vi "TEST_Menu.vi"() -> ()   [LabVIEW 2021]
uses:
  <vilib>/Utility/miscctls.llb/LVMenuShortCut.ctl
  Menu.lvclass
  MenuSelection.ctl
  Picture2D/src/Color/Color.lvclass
  Picture2D/src/2DPictureControl/2DPictureControl.lvclass
  <vilib>/Utility/miscctls.llb/LVPointTypeDef.ctl
  91be992c-c2ba-4221-a176-dbd6ab68e1f9.vi
  Picture2D/src/Picture/Image.lvclass
  C:/GitHub/Picture2D/src/IDrawable/IDrawable.lvclass
  SetBackgroundColor.vi
  SetBorderColor.vi
  SetHiliteColor.vi
  SetHiliteTextColor.vi
  SetTextColor.vi
  <vilib>/ErrorRing/Error Ring.xnode
panel:
  out "enabled":bool
  out "2D Picture out":picture
  in  "Color Theme":enum16{"LabVIEW", "Dark"}(ring)
  out "item name":string
  out "submenu tags":string[](array[string])
  out "checked":bool
  out "short cut":T1
  out "2D Picture":picture
  out "ItemPath":string
  out "ItemTag":string
  out "error out":errorcluster
  out "item tags out":string[](array[string])
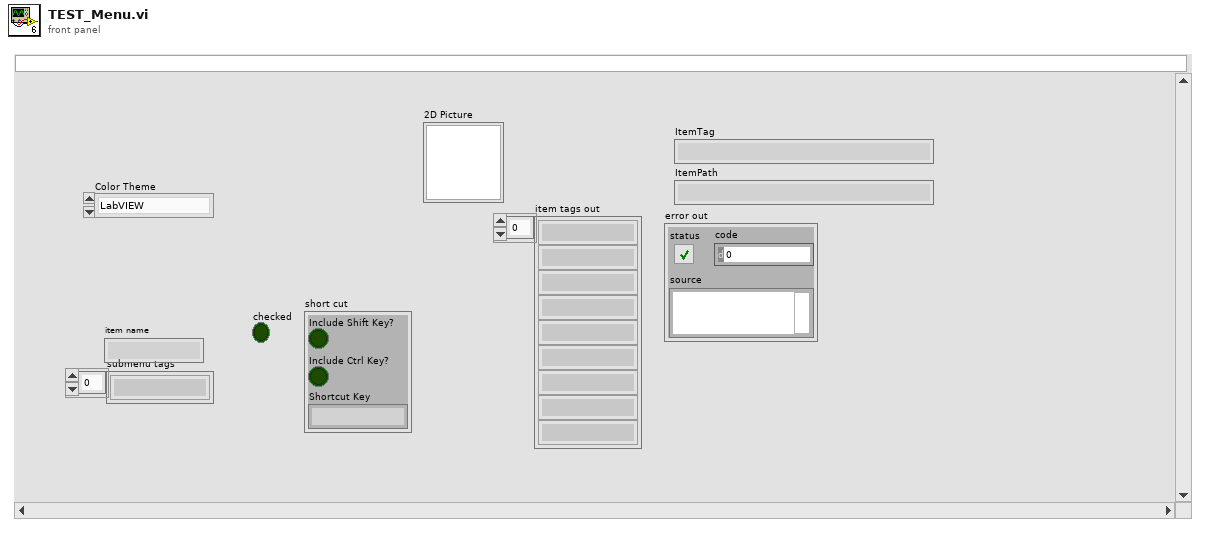
[diagram p1: front panel]
types:
  T1 = typedef "LVMenuShortCut.ctl" = cluster{"Include Shift Key?":bool, "Include Ctrl Key?":bool, "Shortcut Key":string}
  T2 = enum16{"Init Menu", "Init Menu Icon", "Execute", "Close"}
  T3 = enum16{"Init Menu", "Init Menu Icon", "Execute", "Close"}[]
  T4 = typedef "LVPointTypeDef.ctl" = cluster{"Horizontal":i16, "Vertical":i16}
  T5 = typedef "LVBoundsTypeDef.ctl" = cluster{"Width":u32, "Height":u32}
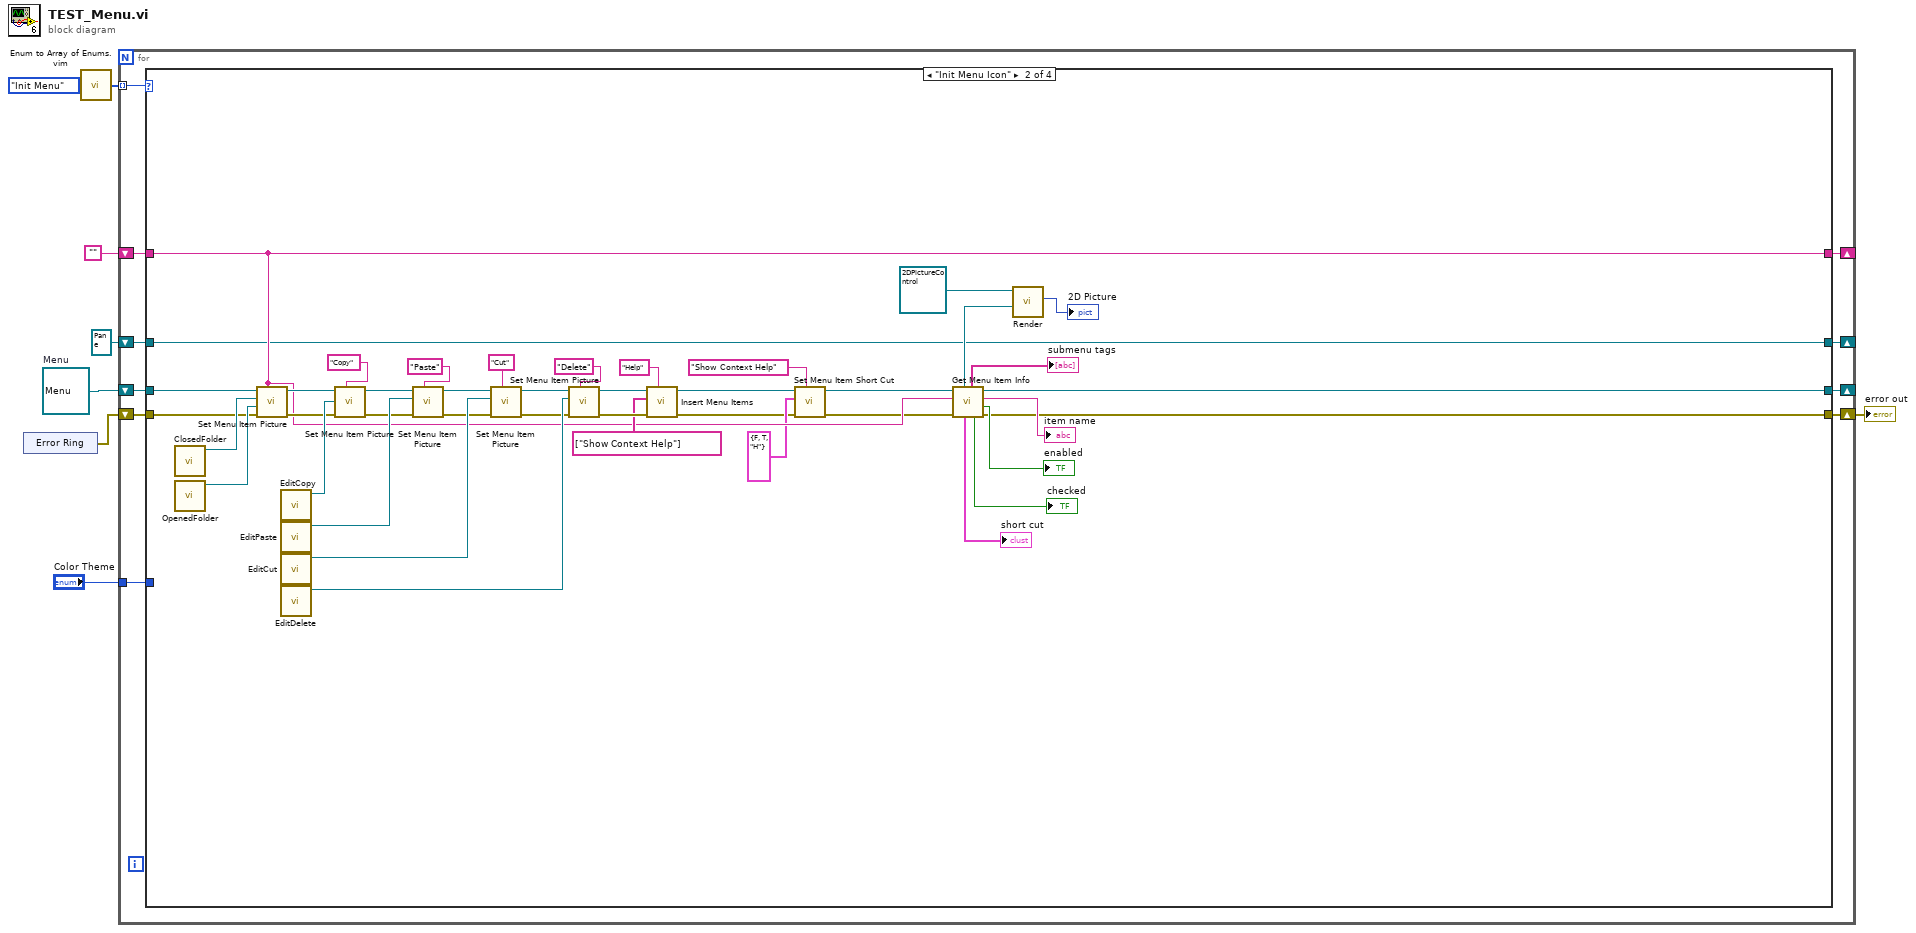
[diagram p0: block diagram]
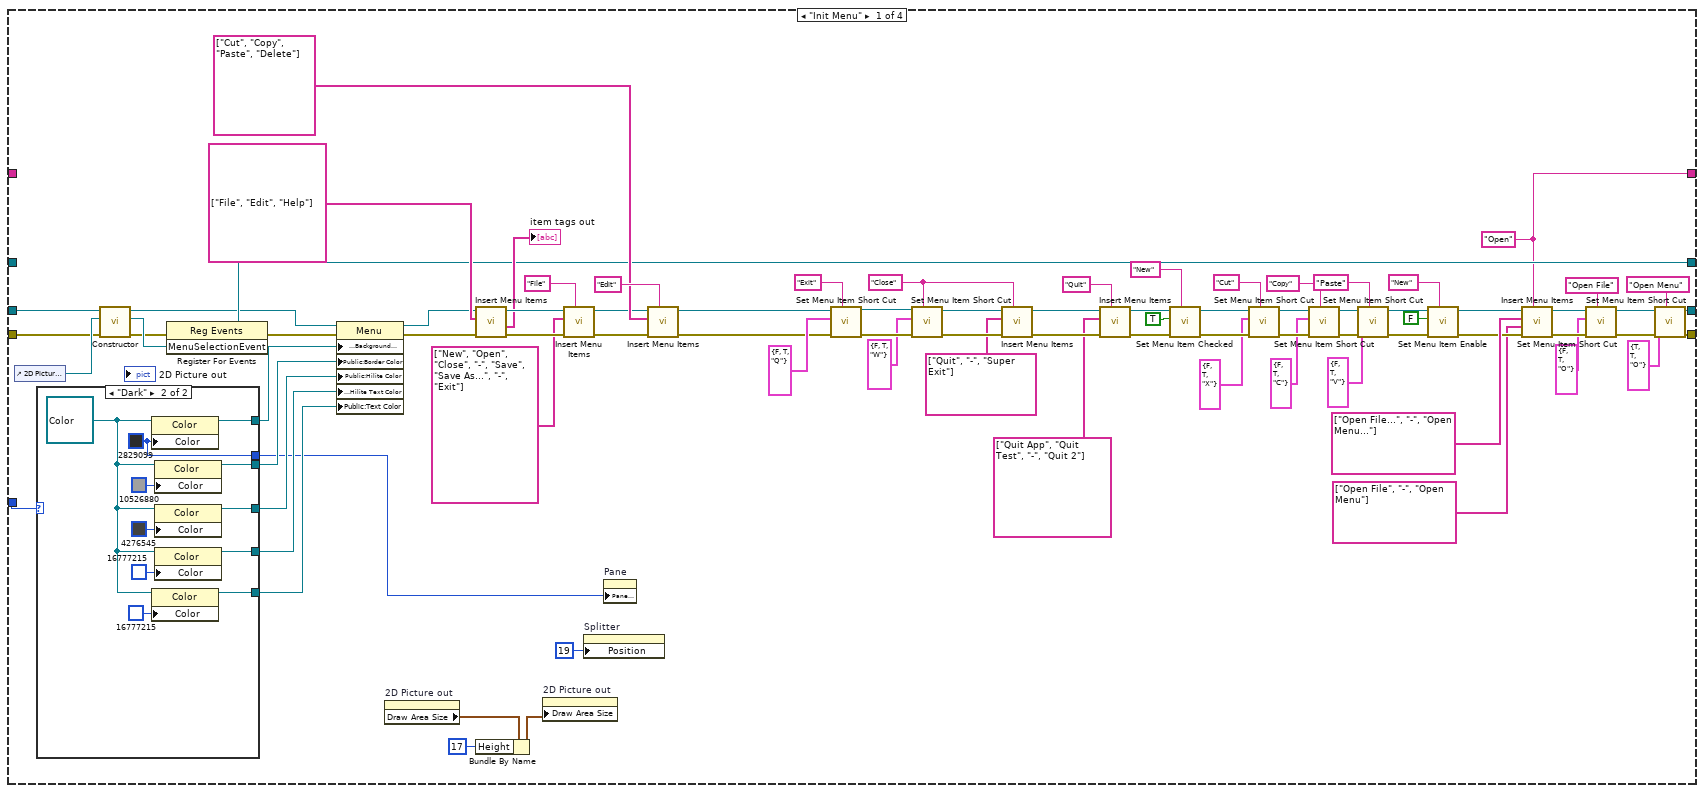
[diagram p2: hidden frame]
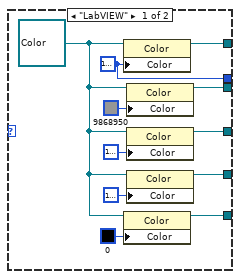
[diagram p3: hidden frame]
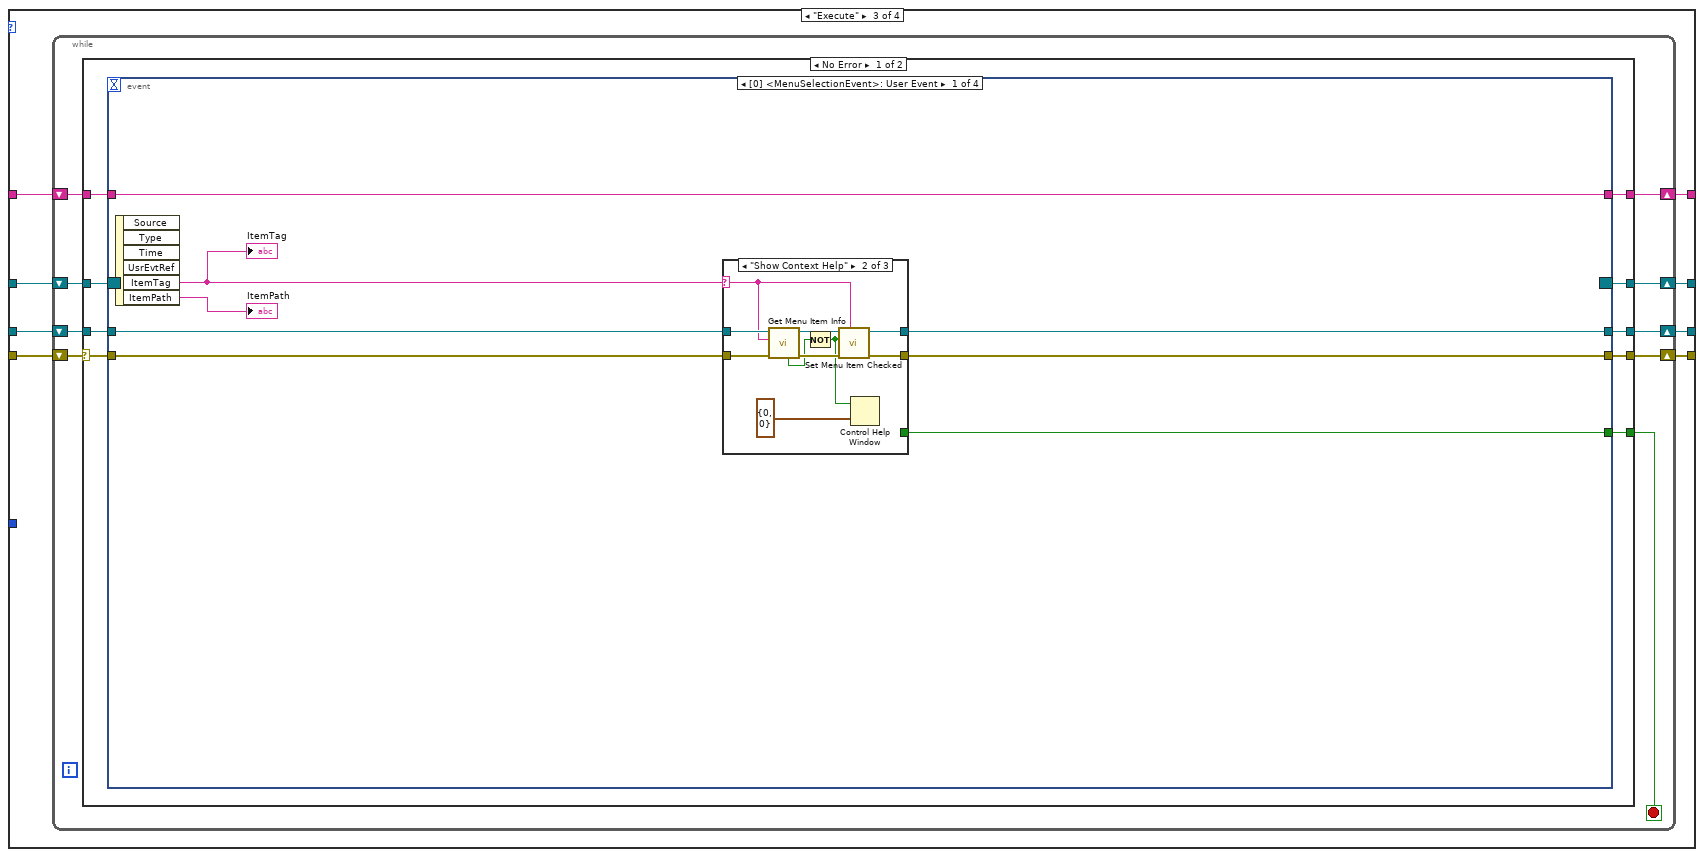
[diagram p4: hidden frame]
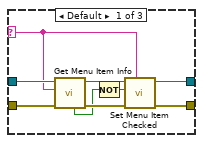
[diagram p5: hidden frame]
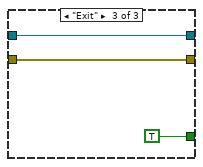
[diagram p6: hidden frame]
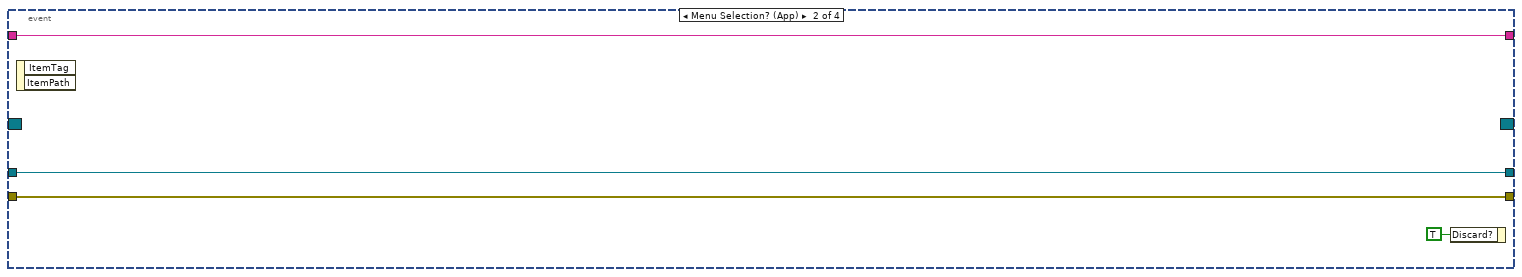
[diagram p7: hidden frame]
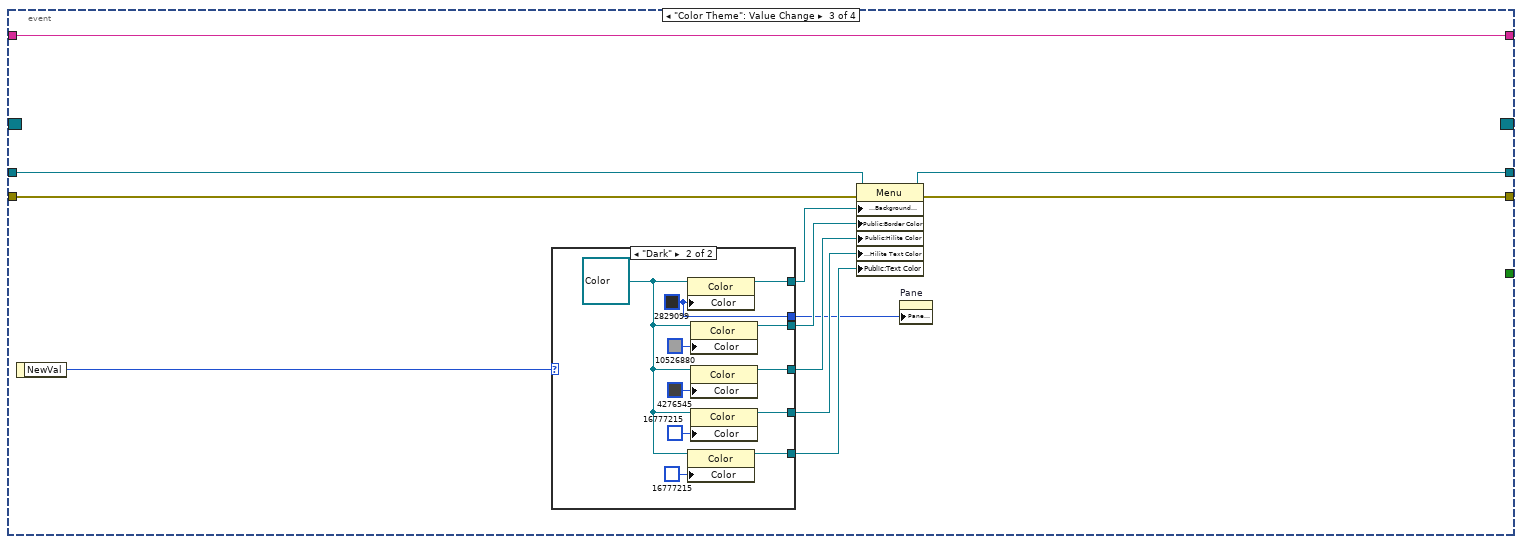
[diagram p8: hidden frame]
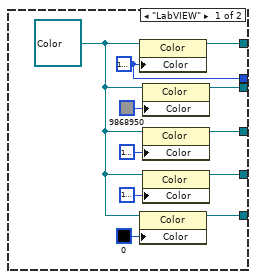
[diagram p9: hidden frame]
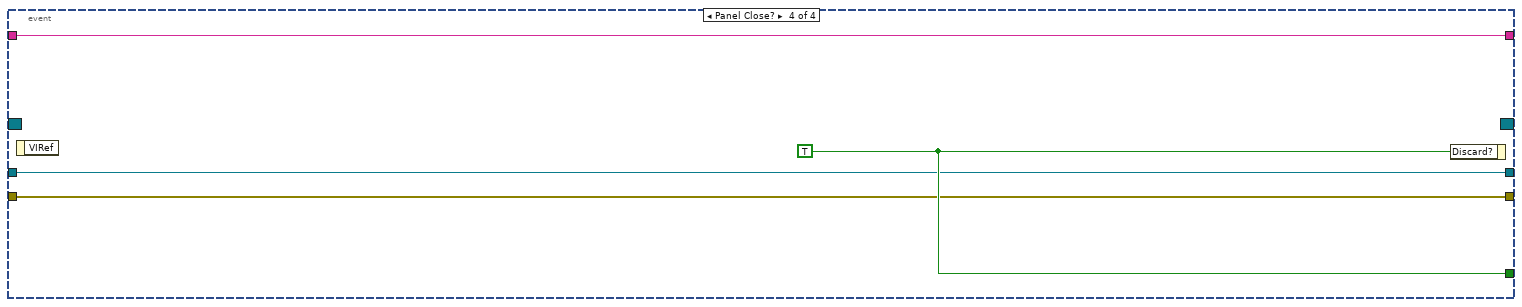
[diagram p10: hidden frame]
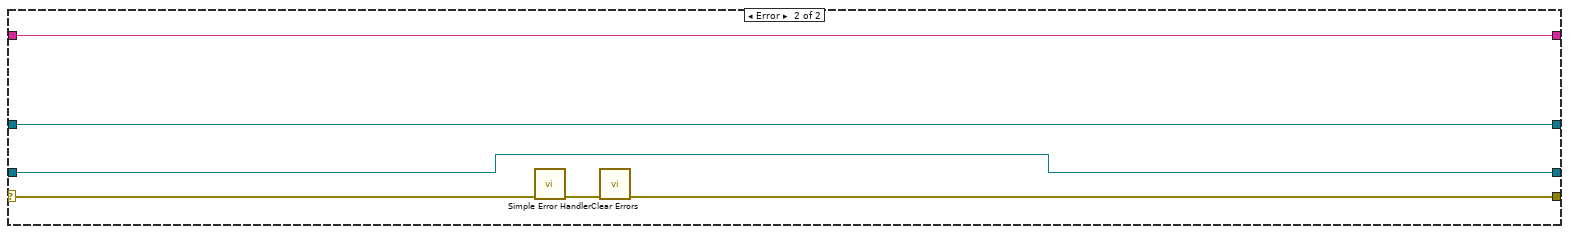
[diagram p11: hidden frame]
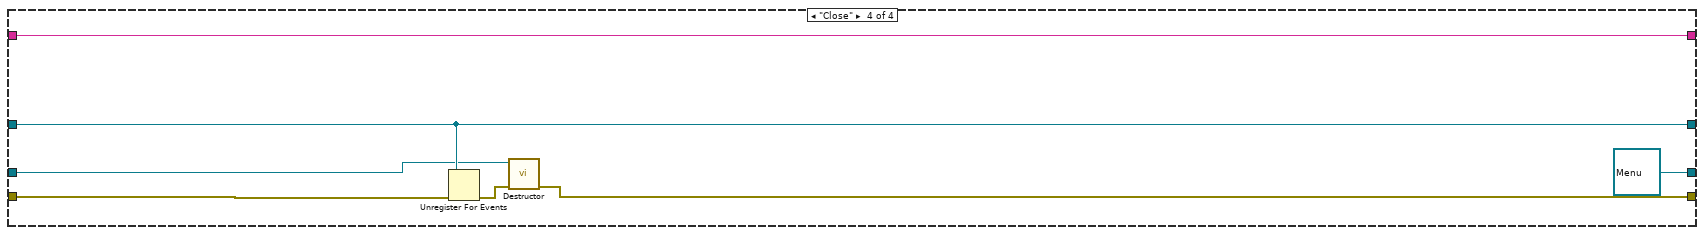
[diagram p12: hidden frame]
diagram:
  w8 = refnum<class "Menu.lvclass"> refnum  # Menu
  n1 = xnode "Error Ring"() -> ("error out"=w4:errorcluster)
  n2 = call "Enum to Array of Enums.vim"("enum"=T2."Init Menu") -> ("array of enums"=w5:T3)
  n3 = for {
    tunnel: "Color Theme" -> [w16]
    shift-right: [w15] -> _
    shift-left: w8 -> [w18]
    tunnel: w5 -> [w12] mode=indexing
    shift-right: [w14] -> w3
    shift-left: w4 -> [w13]
    shift-right: [w17] -> _
    shift-left: refnum<event-registration> refnum ("Event Registration Refnum") -> [w9]
    shift-right: [w11] -> _
    shift-left: "" -> [w10]
    n4 = case shown="\"Init Menu Icon\"" w12 {
      tunnel: w18 -> [w99 w130 w169 w271]
      tunnel: [w73 w131 w170 w273] -> w17
      tunnel: [w67 w132 w164 w269] -> w11
      tunnel: w16 -> [w37 _ _ _]
      tunnel: [w30 w133 w168 refnum<class "Menu.lvclass"> refnum ("Menu")] -> w15
      tunnel: [w29 w134 w167 w272] -> w14
      tunnel: w13 -> [w23 w129 w166 w268]
      tunnel: w10 -> [_ w132 w165 w269]
      tunnel: w9 -> [_ w131 w171 w273]
      frame "Init Menu" {
        w67 = "Open" ("item tag")
        w80 = "Close" ("item tag")
        n5 = control-ref of="2D Picture out"() -> (w74:refnum<vi>)
        n6 = case shown="\"Dark\"" w37 {
          tunnel: [w110 w121] -> w42
          tunnel: [w108 w119] -> w41
          tunnel: [w107 w118] -> w40
          tunnel: [w106 w117] -> w39
          tunnel: [w105 w116] -> w38
          tunnel: [w100 w111] -> w36
          frame "LabVIEW" {
            w100 = u32 16777238 ("Color")
            w109 = refnum<class "Color.lvclass"> refnum ("Background Color")
            n7 = property class="Color"(reference=w109, "Color"=w100) -> (reference out=w110:refnum<class "Color.lvclass">)  [unwired: 1 in, 1 out]
            n8 = property class="Color"(reference=w109, "Color"=u32 0) -> (reference out=w105:refnum<class "Color.lvclass">)  [unwired: 1 in, 1 out]
            n9 = property class="Color"(reference=w109, "Color"=u32 9868950) -> (reference out=w108:refnum<class "Color.lvclass">)  [unwired: 1 in, 1 out]
            n10 = property class="Color"(reference=w109, "Color"=u32 16777224) -> (reference out=w107:refnum<class "Color.lvclass">)  [unwired: 1 in, 1 out]
            n11 = property class="Color"(reference=w109, "Color"=u32 16777226) -> (reference out=w106:refnum<class "Color.lvclass">)  [unwired: 1 in, 1 out]
          }
          frame "Dark" {
            w111 = u32 2829099 ("Color")
            w120 = refnum<class "Color.lvclass"> refnum ("Background Color")
            n12 = property class="Color"(reference=w120, "Color"=w111) -> (reference out=w121:refnum<class "Color.lvclass">)  [unwired: 1 in, 1 out]
            n13 = property class="Color"(reference=w120, "Color"=u32 16777215) -> (reference out=w116:refnum<class "Color.lvclass">)  [unwired: 1 in, 1 out]
            n14 = property class="Color"(reference=w120, "Color"=u32 10526880) -> (reference out=w119:refnum<class "Color.lvclass">)  [unwired: 1 in, 1 out]
            n15 = property class="Color"(reference=w120, "Color"=u32 4276545) -> (reference out=w118:refnum<class "Color.lvclass">)  [unwired: 1 in, 1 out]
            n16 = property class="Color"(reference=w120, "Color"=u32 16777215) -> (reference out=w117:refnum<class "Color.lvclass">)  [unwired: 1 in, 1 out]
          }
        }
        n17 = call "Constructor.vi"("error in (no error)"=w23, "PictRef"=w74, "Menu in"=w99) -> ("error out"=w89:errorcluster, "MenuSelectionEvent"=w91:refnum<user-event>, "Menu out"=w44:refnum<class "Menu.lvclass">)  [unwired: 6 in]
        n18 = register-events(error in=w89, w91) -> (reference out=w73:refnum<event-registration>, error out=w90:errorcluster)  [unwired: 1 in]
        n19 = property class="Menu"(reference=w44, error in=w90, "Public:Background Color"=w42, "Public:Border Color"=w41, "Public:Hilite Color"=w40, "Public:Hilite Text Color"=w39, "Public:Text Color"=w38) -> (reference out=w43:refnum<class "Menu.lvclass">, error out=w45:errorcluster)
        n20 = property on="2D Picture out" class="Pict"() -> ("Draw Area Size"=w21:T5)  [unwired: 2 in, 2 out]
        n21 = call "Insert Menu Items.vi"("error in (no error)"=w45, "item names"=string[] ["File", "Edit", "Help"], "Menu in"=w43) -> ("error out"=w96:errorcluster, "item tags out"=→"item tags out":string[], "Menu out"=w97:refnum<class "Menu.lvclass">)  [unwired: 6 in]
        n22 = Bundle By Name(cluster=w21, "Height"=u32 17) -> (w20:T5)
        n23 = property on="2D Picture out" class="Pict"("Draw Area Size"=w20) -> ()  [unwired: 2 in, 2 out]
        n24 = call "Insert Menu Items.vi"("menu tag"="File", "error in (no error)"=w96, "item names"=string[] ["New", "Open", "Close", "-", "Save", "Save As...", "-", "Exit"], "Menu in"=w97) -> ("error out"=w47:errorcluster, "Menu out"=w49:refnum<class "Menu.lvclass">)  [unwired: 5 in, 1 out]
        n25 = property on="Splitter" class="Splitter"("Position"=19 ("Splitter Position")) -> ()  [unwired: 2 in, 2 out]
        n26 = property on="Pane" class="Pane"("PaneColor"=w36) -> ()  [unwired: 2 in, 2 out]
        n27 = call "Insert Menu Items.vi"("menu tag"="Edit", "error in (no error)"=w47, "item names"=string[] ["Cut", "Copy", "Paste", "Delete"], "Menu in"=w49) -> ("error out"=w46:errorcluster, "Menu out"=w48:refnum<class "Menu.lvclass">)  [unwired: 5 in, 1 out]
        n28 = call "Set Menu Item Short Cut.vi"("item tag"="Exit", "error in (no error)"=w46, "short cut"=T1 {"Include Shift Key?"=FALSE, "Include Ctrl Key?"=TRUE, "Shortcut Key"="Q"}, "Menu in"=w48) -> ("error out"=w85:errorcluster, "Menu out"=w84:refnum<class "Menu.lvclass">)  [unwired: 6 in]
        n29 = call "Set Menu Item Short Cut.vi"("item tag"=w80, "error in (no error)"=w85, "short cut"=T1 {"Include Shift Key?"=FALSE, "Include Ctrl Key?"=TRUE, "Shortcut Key"="W"}, "Menu in"=w84) -> ("error out"=w81:errorcluster, "Menu out"=w82:refnum<class "Menu.lvclass">)  [unwired: 6 in]
        n30 = call "Insert Menu Items.vi"("menu tag"=w80, "error in (no error)"=w81, "item names"=string[] ["Quit", "-", "Super Exit"], "Menu in"=w82) -> ("error out"=w77:errorcluster, "Menu out"=w76:refnum<class "Menu.lvclass">)  [unwired: 5 in, 1 out]
        n31 = call "Insert Menu Items.vi"("menu tag"="Quit", "error in (no error)"=w77, "item names"=string[] ["Quit App", "Quit Test", "-", "Quit 2"], "Menu in"=w76) -> ("error out"=w71:errorcluster, "Menu out"=w72:refnum<class "Menu.lvclass">)  [unwired: 5 in, 1 out]
        n32 = call "Set Menu Item Checked.vi"("item tag"="New", "error in (no error)"=w71, "checked"=TRUE, "Menu in"=w72) -> ("error out"=w65:errorcluster, "Menu out"=w66:refnum<class "Menu.lvclass">)  [unwired: 6 in]
        n33 = call "Set Menu Item Short Cut.vi"("item tag"="Cut", "error in (no error)"=w65, "short cut"=T1 {"Include Shift Key?"=FALSE, "Include Ctrl Key?"=TRUE, "Shortcut Key"="X"}, "Menu in"=w66) -> ("error out"=w62:errorcluster, "Menu out"=w61:refnum<class "Menu.lvclass">)  [unwired: 6 in]
        n34 = call "Set Menu Item Short Cut.vi"("item tag"="Copy", "error in (no error)"=w62, "short cut"=T1 {"Include Shift Key?"=FALSE, "Include Ctrl Key?"=TRUE, "Shortcut Key"="C"}, "Menu in"=w61) -> ("error out"=w64:errorcluster, "Menu out"=w63:refnum<class "Menu.lvclass">)  [unwired: 6 in]
        n35 = call "Set Menu Item Short Cut.vi"("item tag"="Paste", "error in (no error)"=w64, "short cut"=T1 {"Include Shift Key?"=FALSE, "Include Ctrl Key?"=TRUE, "Shortcut Key"="V"}, "Menu in"=w63) -> ("error out"=w55:errorcluster, "Menu out"=w53:refnum<class "Menu.lvclass">)  [unwired: 6 in]
        n36 = call "Set Menu Item Enable.vi"("item tag"="New", "error in (no error)"=w55, "enabled"=FALSE, "Menu in"=w53) -> ("error out"=w54:errorcluster, "Menu out"=w52:refnum<class "Menu.lvclass">)  [unwired: 6 in]
        n37 = call "Insert Menu Items.vi"("menu tag"=w67, "error in (no error)"=w54, "item tags"=string[] ["Open File", "-", "Open Menu"] ("item names"), "item names"=string[] ["Open File...", "-", "Open Menu..."], "Menu in"=w52) -> ("error out"=w33:errorcluster, "Menu out"=w34:refnum<class "Menu.lvclass">)  [unwired: 4 in, 1 out]
        n38 = call "Set Menu Item Short Cut.vi"("item tag"="Open File", "error in (no error)"=w33, "short cut"=T1 {"Include Shift Key?"=FALSE, "Include Ctrl Key?"=TRUE, "Shortcut Key"="O"}, "Menu in"=w34) -> ("error out"=w32:errorcluster, "Menu out"=w31:refnum<class "Menu.lvclass">)  [unwired: 6 in]
        n39 = call "Set Menu Item Short Cut.vi"("item tag"="Open Menu", "error in (no error)"=w32, "short cut"=T1 {"Include Shift Key?"=TRUE, "Include Ctrl Key?"=TRUE, "Shortcut Key"="O"}, "Menu in"=w31) -> ("error out"=w29:errorcluster, "Menu out"=w30:refnum<class "Menu.lvclass">)  [unwired: 6 in]
      }
      frame "Init Menu Icon" {
        n40 = call "ClosedFolder.vi"() -> ("Image out"=w162:refnum<class "Image.lvclass">)  [unwired: 11 in]
        n41 = call "OpenedFolder.vi"() -> ("Image out"=w163:refnum<class "Image.lvclass">)  [unwired: 11 in]
        n42 = call "Set Menu Item Picture.vi"("item tag"=w132, "error in (no error)"=w129, "Hilite Picture"=w163, "Picture"=w162, "Menu in"=w130) -> ("error out"=w149:errorcluster, "Menu out"=w148:refnum<class "Menu.lvclass">)  [unwired: 5 in]
        n43 = call "EditCopy.vi"() -> ("Image out"=w158:refnum<class "Image.lvclass">)  [unwired: 11 in]
        n44 = call "EditPaste.vi"() -> ("Image out"=w159:refnum<class "Image.lvclass">)  [unwired: 11 in]
        n45 = call "EditCut.vi"() -> ("Image out"=w160:refnum<class "Image.lvclass">)  [unwired: 11 in]
        n46 = call "EditDelete.vi"() -> ("Image out"=w161:refnum<class "Image.lvclass">)  [unwired: 11 in]
        n47 = call "Set Menu Item Picture.vi"("item tag"="Copy", "error in (no error)"=w149, "Picture"=w158, "Menu in"=w148) -> ("error out"=w151:errorcluster, "Menu out"=w150:refnum<class "Menu.lvclass">)  [unwired: 6 in]
        n48 = call "Set Menu Item Picture.vi"("item tag"="Paste", "error in (no error)"=w151, "Picture"=w159, "Menu in"=w150) -> ("error out"=w153:errorcluster, "Menu out"=w152:refnum<class "Menu.lvclass">)  [unwired: 6 in]
        n49 = call "Set Menu Item Picture.vi"("item tag"="Cut", "error in (no error)"=w153, "Picture"=w160, "Menu in"=w152) -> ("error out"=w155:errorcluster, "Menu out"=w154:refnum<class "Menu.lvclass">)  [unwired: 6 in]
        n50 = call "Set Menu Item Picture.vi"("item tag"="Delete", "error in (no error)"=w155, "Picture"=w161, "Menu in"=w154) -> ("error out"=w157:errorcluster, "Menu out"=w156:refnum<class "Menu.lvclass">)  [unwired: 6 in]
        n51 = call "Insert Menu Items.vi"("menu tag"="Help", "error in (no error)"=w157, "item names"=string[] ["Show Context Help"], "Menu in"=w156) -> ("error out"=w127:errorcluster, "Menu out"=w125:refnum<class "Menu.lvclass">)  [unwired: 5 in, 1 out]
        n52 = call "Set Menu Item Short Cut.vi"("item tag"="Show Context Help", "error in (no error)"=w127, "short cut"=T1 {"Include Shift Key?"=FALSE, "Include Ctrl Key?"=TRUE, "Shortcut Key"="H"}, "Menu in"=w125) -> ("error out"=w126:errorcluster, "Menu out"=w124:refnum<class "Menu.lvclass">)  [unwired: 6 in]
        n53 = call "Get Menu Item Info.vi"("error in (no error)"=w126, "item tag"=w132, "Menu in"=w124) -> ("error out"=w134:errorcluster, "enabled"=→"enabled":bool, "item name"=→"item name":string, "Menu out"=w133:refnum<class "Menu.lvclass">, "checked"=→"checked":bool, "submenu tags"=→"submenu tags":string[], "short cut"=→"short cut":T1, "Picture"=w136:refnum<class "Image.lvclass">)  [unwired: 1 in]
        n54 = call-dynamic "Render.vi"("IDrawable"=w136, "2DPictureControl in"=refnum<class "2DPictureControl.lvclass"> refnum) -> ("2D Picture out"=→"2D Picture":picture)  [unwired: 7 in, 2 out]
      }
      frame "Execute" {
        n55 = while {
          shift-right: [w178] -> w167
          shift-left: w166 -> [w179]
          shift-right: [w175] -> w170
          shift-left: w171 -> [w180]
          shift-right: [w176] -> w168
          shift-left: w169 -> [w177]
          shift-right: [w172] -> w164
          shift-left: w165 -> [w173]
          stop <- w174 stop-if-true
          n56 = case shown="No Error" w179 {
            selector: w179 -> [w188 w267]
            tunnel: w180 -> [w189 w266]
            tunnel: [w187 w263] -> w178
            tunnel: w177 -> [w186 w265]
            tunnel: [w185 w265] -> w176
            tunnel: [w184 w266] -> w175
            tunnel: [w183 _] -> w174
            tunnel: w173 -> [w182 w262]
            tunnel: [w181 w262] -> w172
            frame No Error {
              n57 = event shown="[0] <MenuSelectionEvent>: User Event" {
                selector: w189 -> [_ _ _ _]
                dyn-events: [_ _ _ _] -> w184
                timeout: _ -> [_ _ _ _]
                tunnel: [w192 w223 w226 w260] -> w187
                tunnel: w188 -> [w193 w223 w229 w260]
                tunnel: [w191 w222 w225 w259] -> w185
                tunnel: w186 -> [w194 w222 w228 w259]
                tunnel: [w195 _ _ w261] -> w183
                tunnel: w182 -> [w190 w221 w224 w258]
                tunnel: [w190 w221 w224 w258] -> w181
                event User Event {
                  n58 = event-data() -> ("ItemTag"=w196:string, "ItemPath"=→"ItemPath":string)  [unwired: 1 in, 4 out]
                  "ItemTag" <- w196
                  n59 = case shown="\"Show Context Help\"" w196 {
                    selector: w196 -> [w198 w210 _]
                    tunnel: [_ _ TRUE] -> w195
                    tunnel: w194 -> [w206 w216 w218]
                    tunnel: w193 -> [w205 w215 w217]
                    tunnel: [w203 w213 w217] -> w192
                    tunnel: [w201 w211 w218] -> w191
                    frame Default {
                      n60 = call "Get Menu Item Info.vi"("error in (no error)"=w205, "item tag"=w198, "Menu in"=w206) -> ("error out"=w204:errorcluster, "Menu out"=w202:refnum<class "Menu.lvclass">, "checked"=w200:bool)  [unwired: 1 in, 5 out]
                      n61 = Not(x=w200) -> (.not. x?=w199:bool)
                      n62 = call "Set Menu Item Checked.vi"("item tag"=w198, "error in (no error)"=w204, "checked"=w199, "Menu in"=w202) -> ("error out"=w203:errorcluster, "Menu out"=w201:refnum<class "Menu.lvclass">)  [unwired: 6 in]
                    }
                    frame "Show Context Help" {
                      n63 = call "Get Menu Item Info.vi"("error in (no error)"=w215, "item tag"=w210, "Menu in"=w216) -> ("error out"=w214:errorcluster, "Menu out"=w212:refnum<class "Menu.lvclass">, "checked"=w208:bool)  [unwired: 1 in, 5 out]
                      n64 = Not(x=w208) -> (.not. x?=w207:bool)
                      n65 = call "Set Menu Item Checked.vi"("item tag"=w210, "error in (no error)"=w214, "checked"=w207, "Menu in"=w212) -> ("error out"=w213:errorcluster, "Menu out"=w211:refnum<class "Menu.lvclass">)  [unwired: 6 in]
                      n66 = Control Help Window(0:T4 {"Horizontal"=0, "Vertical"=0} ("Top Left Corner"), 1:w207) -> ()
                    }
                    frame "Exit" {
                    }
                  }
                }
                event Menu Selection? (App) {
                  n67 = event-data() -> ()  [unwired: 1 in, 2 out]
                  n68 = event-data("Discard?"=TRUE) -> ()  [unwired: 1 in, 1 out]
                }
                event "Color Theme": Value Change {
                  n69 = event-data() -> ("NewVal"=w230:enum16{"LabVIEW", "Dark"})  [unwired: 1 in]
                  n70 = case shown="\"Dark\"" w230 {
                    tunnel: [w246 w257] -> w235
                    tunnel: [w244 w255] -> w234
                    tunnel: [w243 w254] -> w233
                    tunnel: [w242 w253] -> w232
                    tunnel: [w241 w252] -> w231
                    tunnel: [w236 w247] -> w227
                    frame "LabVIEW" {
                      w236 = u32 16777238 ("Color")
                      w245 = refnum<class "Color.lvclass"> refnum ("Background Color")
                      n71 = property class="Color"(reference=w245, "Color"=w236) -> (reference out=w246:refnum<class "Color.lvclass">)  [unwired: 1 in, 1 out]
                      n72 = property class="Color"(reference=w245, "Color"=u32 0) -> (reference out=w241:refnum<class "Color.lvclass">)  [unwired: 1 in, 1 out]
                      n73 = property class="Color"(reference=w245, "Color"=u32 9868950) -> (reference out=w244:refnum<class "Color.lvclass">)  [unwired: 1 in, 1 out]
                      n74 = property class="Color"(reference=w245, "Color"=u32 16777224) -> (reference out=w243:refnum<class "Color.lvclass">)  [unwired: 1 in, 1 out]
                      n75 = property class="Color"(reference=w245, "Color"=u32 16777226) -> (reference out=w242:refnum<class "Color.lvclass">)  [unwired: 1 in, 1 out]
                    }
                    frame "Dark" {
                      w247 = u32 2829099 ("Color")
                      w256 = refnum<class "Color.lvclass"> refnum ("Background Color")
                      n76 = property class="Color"(reference=w256, "Color"=w247) -> (reference out=w257:refnum<class "Color.lvclass">)  [unwired: 1 in, 1 out]
                      n77 = property class="Color"(reference=w256, "Color"=u32 16777215) -> (reference out=w252:refnum<class "Color.lvclass">)  [unwired: 1 in, 1 out]
                      n78 = property class="Color"(reference=w256, "Color"=u32 10526880) -> (reference out=w255:refnum<class "Color.lvclass">)  [unwired: 1 in, 1 out]
                      n79 = property class="Color"(reference=w256, "Color"=u32 4276545) -> (reference out=w254:refnum<class "Color.lvclass">)  [unwired: 1 in, 1 out]
                      n80 = property class="Color"(reference=w256, "Color"=u32 16777215) -> (reference out=w253:refnum<class "Color.lvclass">)  [unwired: 1 in, 1 out]
                    }
                  }
                  n81 = property class="Menu"(reference=w228, error in=w229, "Public:Background Color"=w235, "Public:Border Color"=w234, "Public:Hilite Color"=w233, "Public:Hilite Text Color"=w232, "Public:Text Color"=w231) -> (reference out=w225:refnum<class "Menu.lvclass">, error out=w226:errorcluster)
                  n82 = property on="Pane" class="Pane"("PaneColor"=w227) -> ()  [unwired: 2 in, 2 out]
                }
                event Panel Close? {
                  w261 = TRUE ("Discard?")
                  n83 = event-data() -> ()  [unwired: 1 in, 1 out]
                  n84 = event-data("Discard?"=w261) -> ()  [unwired: 1 in, 1 out]
                }
              }
            }
            frame Error {
              n85 = call <vilib>:"Simple Error Handler.vi"("error in (no error)"=w267) -> ("error out"=w264:errorcluster)  [unwired: 4 in, 4 out]
              n86 = call <vilib>:"Clear Errors.vi"("error in (no error)"=w264) -> ("error out"=w263:errorcluster)  [unwired: 5 in, 1 out]
            }
          }
        }
      }
      frame "Close" {
        n87 = Unregister For Events(event registration refnum=w273, error in=w268) -> (error out=w274:errorcluster)
        n88 = call "Destructor.vi"("error in (no error)"=w274, "Menu in"=w271) -> ("error out"=w272:errorcluster)  [unwired: 9 in]
      }
    }
  }
  "error out" <- w3
